vi "Configure Trigger Source [TRG].vi"(8 "error in (no error)":errorcluster, 9 "source (Immediate)":i32(ring) items=["Immediate", "External", "Software", "TTL0", "TTL1", "TTL2", "TTL3", "TTL4", "TTL5", "TTL6", "TTL7", "ECL0", "ECL1", "PXI Star", "RTSI 0", "RTSI 1", "RTSI 2", "RTSI 3", "RTSI 4", "RTSI 5", "RTSI 6"], 10 "channel name (\"CHANNEL1\")":string="CHANNEL1", 11 "CS++DCPwr in":refnum<class "CS++DCPwr.lvclass">) -> (0 "error out":errorcluster, 3 "CS++DCPwr out":refnum<class "CS++DCPwr.lvclass">)   [LabVIEW 2016, in "CS++DCPwr.lvlib" / "CS++DCPwr.lvclass"]
doc: "This VI configures the trigger source to which the power supply responds after you call IviDCPwr Initiate [TRG]. When the power supply receives a trigger signal on the source you specify, it changes its current and voltage outputs.\n\nYou configure the triggered current and voltage outputs with the\nIviDCPwr Configure Triggered Current Limit [TRG] and \nIviDCPwr Configure Triggered Voltage Level [TRG] VIs. \n\nNotes:\n\n(1) This VI is part of the IviDCPwrTrigger [TRG] extension group."
uses:
  CS++DCPwr.lvclass
  CSPP_Core/Classes/CS++ProcessVariables/ProcessVariable/PV.lvclass
  PV-Enum.ctl
  CSPP_Core/Classes/CS++ProcessVariables/ProcessVariable/PV.lvclass/PV.ctl
  CS++DCPwr.lvclass/CS++DCPwr.ctl
  CSPP_Core/Classes/CS++ProcessVariables/ProcessVariable/Write Data.vi
  CSPP_Core/Classes/CS++ProcessVariables/ProcessVariable/Write Timestamp.vi
  CSPP_Core/Classes/CS++ProcessVariables/ProcessVariable/Write Quality.vi
  CSPP_Core/Classes/CS++ProcessVariables/ProcessVariable/Write status.vi
  CSPP_Core/Classes/CS++ProcessVariables/PVConnection/PVConnection.lvclass
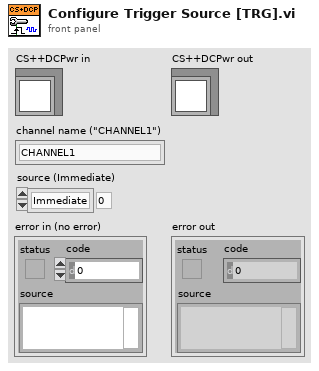
[diagram p1: front panel]
types:
  T1 = typedef "CS++DCPwr.lvlib/CS++DCPwr.lvclass/PV-Enum.ctl" = enum16{"CurrentLimit", "MaxCurrentLimit", "MaxVoltageLevel", "Measure-A", "Measure-V", "OVPLimit", "Range", "TriggerCurrentLimit", "TriggerVoltageLevel", "VoltageLevel", "Behavior", "DesiredOutputState", "RangeType", "TriggerSource", "InState", "OutputEnable", "OVPEnabled"}
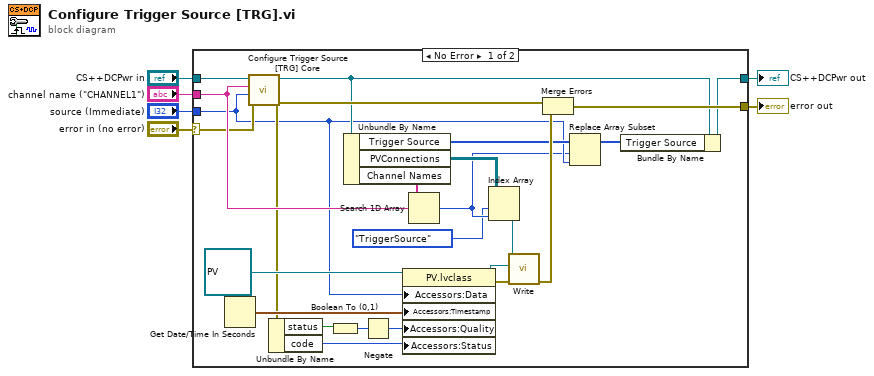
[diagram p0: block diagram]
diagram:
  n1 = case shown="No Error" "error in (no error)" {
    selector: "error in (no error)" -> [w10 w31]
    tunnel: "CS++DCPwr in" -> [w30 w32]
    tunnel: "source (Immediate)" -> [w9 _]
    tunnel: "channel name (\"CHANNEL1\")" -> [w17 _]
    tunnel: [w15 w31] -> w1
    tunnel: [w13 w32] -> w2
    frame No Error {
      n2 = Get Date/Time In Seconds() -> (seconds since 1Jan1904=w29:timestamp)
      n3 = call-dynamic "Configure Trigger Source [TRG] Core.vi"("error in (no error)"=w10, "source (Immediate)"=w9, "channel name (\"CHANNEL1\")"=w17, "CS++DCPwr in"=w30) -> ("error out"=w16:errorcluster, "CS++DCPwr out"=w14:refnum<class "CS++DCPwr.lvclass">)  [unwired: 6 in]
      n4 = Unbundle By Name(w16) -> ("status"=w21:bool, "code"=w19:i32)
      n5 = Boolean To (0,1)(Boolean=w21) -> (0, 1=w20:i16)
      n6 = Unbundle By Name(w14) -> ("Trigger Source"=w12:i32[], "PVConnections"=w24:refnum<class "PVConnection.lvclass">[][], "Channel Names"=w25:string[])
      n7 = Negate(x=w20) -> (-x=w18:i16)
      n8 = property class="PV.lvclass"(reference=refnum<class "PV.lvclass"> refnum ("PV"), "Accessors:Data"=w9, "Accessors:Timestamp"=w29, "Accessors:Quality"=w18, "Accessors:Status"=w19) -> (reference out=w26:refnum<class "PV.lvclass">, error out=w27:errorcluster)  [unwired: 1 in]
      n9 = Search 1D Array(1D array=w25, element=w17) -> (index of element=w8:i32)  [unwired: 1 in]
      n10 = Index Array(array=w24, index (row)=PV-Enum."TriggerSource" ("PV-Enum"), index (col)=w8) -> (element=w23:refnum<class "PVConnection.lvclass">)
      n11 = call "Write.vi"("error in (no error)"=w27, "PV"=w26, "PVConnection in"=w23) -> ("error out"=w22:errorcluster)  [unwired: 7 in, 1 out]
      n12 = Merge Errors(w16, w22) -> (w15:errorcluster)
      n13 = Replace Array Subset(array=w12, new element=w9, index=w8) -> (w11:i32[])
      n14 = Bundle By Name(cluster=w14, "Trigger Source"=w11) -> (w13:refnum<class "CS++DCPwr.lvclass">)
    }
    frame Error {
    }
  }
  "error out" <- w1
  "CS++DCPwr out" <- w2
